vi "SF.vi"(9 "数值输入":i32, 10 "pADStatus":i32[](array[numeric]), 11 "数值 3":i32) -> (3 "数值输出":u32)   [LabVIEW 2012]
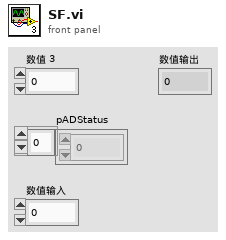
[diagram p1: front panel]
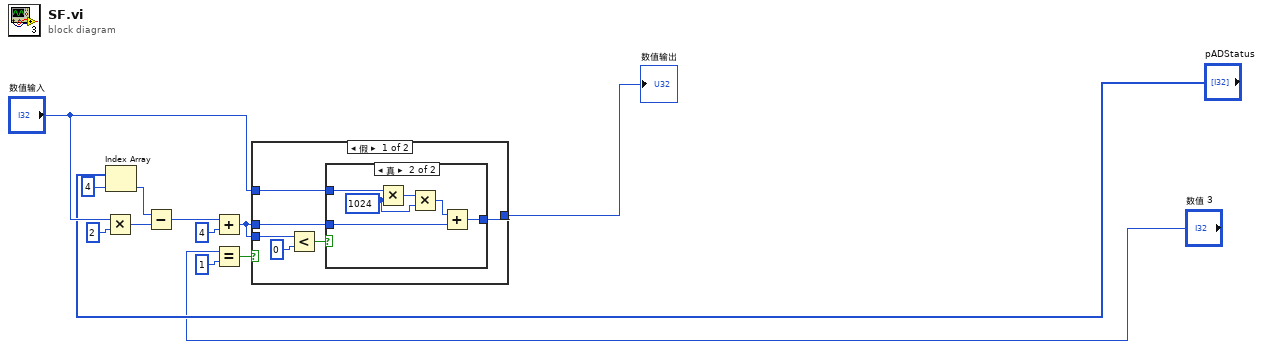
[diagram p0: block diagram]
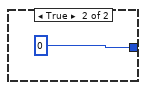
[diagram p3: hidden frame]
diagram:
  n1 = Multiply(x="数值输入", y=u32 2) -> (x*y=w3:u32)
  n2 = Index Array(array="pADStatus", index=4) -> (element=w10:i32)
  n3 = Subtract(x=w10, y=w3) -> (x-y=w1:u32)
  n4 = Add(x=w1, y=u32 4) -> (x+y=w11:u32)
  n5 = Equal?(x="数值 3", y=u32 1) -> (x = y?=w5:bool)
  n6 = case shown="假" w5 {
    tunnel: [w15 u32 0] -> w8
    tunnel: w11 -> [w18 _]
    tunnel: w11 -> [w16 _]
    tunnel: "数值输入" -> [w14 _]
    frame False {
      n7 = Less?(x=w18, y=u32 0) -> (x < y?=w17:bool)
      n8 = case shown="真" w17 {
        tunnel: w16 -> [w20 w24]
        tunnel: [w20 w23] -> w15
        tunnel: w14 -> [_ w22]
        frame False {
        }
        frame True {
          w21 = u32 1024
          n9 = Multiply(x=w22, y=w21) -> (x*y=w26:u32)
          n10 = Multiply(x=w26, y=w21) -> (x*y=w25:u32)
          n11 = Add(x=w25, y=w24) -> (x+y=w23:u32)
        }
      }
    }
    frame True {
    }
  }
  "数值输出" <- w8
